vi "SA40144C.20201230 Data Analysis.vi"() -> ()   [LabVIEW 2020]
uses:
  <vilib>/Analysis/baseanly.llb/Mean (DBL).vi
  <userlib>/_OpenG.lib/file/file.llb/Build Path - Traditional__ogtk.vi
  <userlib>/LevyLab/LV to ITX/Data/Data.lvclass
  <vilib>/Analysis/NI_AALBase.lvlib
  <userlib>/LevyLab/XY Utilities/xy_utilities.lvlib
panel:
  out "Temp vs t":T1(graph)
  in  "Update":bool
  in  "Temps to keep (Lifespan)":i32=26
  in  "Temps to keep (Arrhenius fit)":i32=26
  out "E_a":dbl[](array[numeric])
  in  "Trimming":i32=400
  out "G4T vs t  2D":T1(graph)
  out "G2T vs t 2D":T1(graph)
  in  "Data File":path=path "G:/My Drive/ansom/Data/PPMS 2/SA40144C.20201230/01 - Temp Sweep 1 HR/SA40144C.20201230.275K.dat"
  in  "Final Temp":i32=400
  in  "Temp Step":i32=5
  in  "Init Temp":i32=275
  in  "Source Voltage":dbl=0.01
  in  "OK":bool
  out "error out":errorcluster
  in  "error in (no error)":errorcluster
  out "G4T vs t":T1(graph)
  out "Arrhenius":T1(graph)
  out "Lifespan vs Temp (hrs)":cluster{i32[], dbl[]}[](graph)
  out "G2T vs t":T1(graph)
  # "2T"
  # "4T"
  # "2T 2D"
  # "4T 2D"
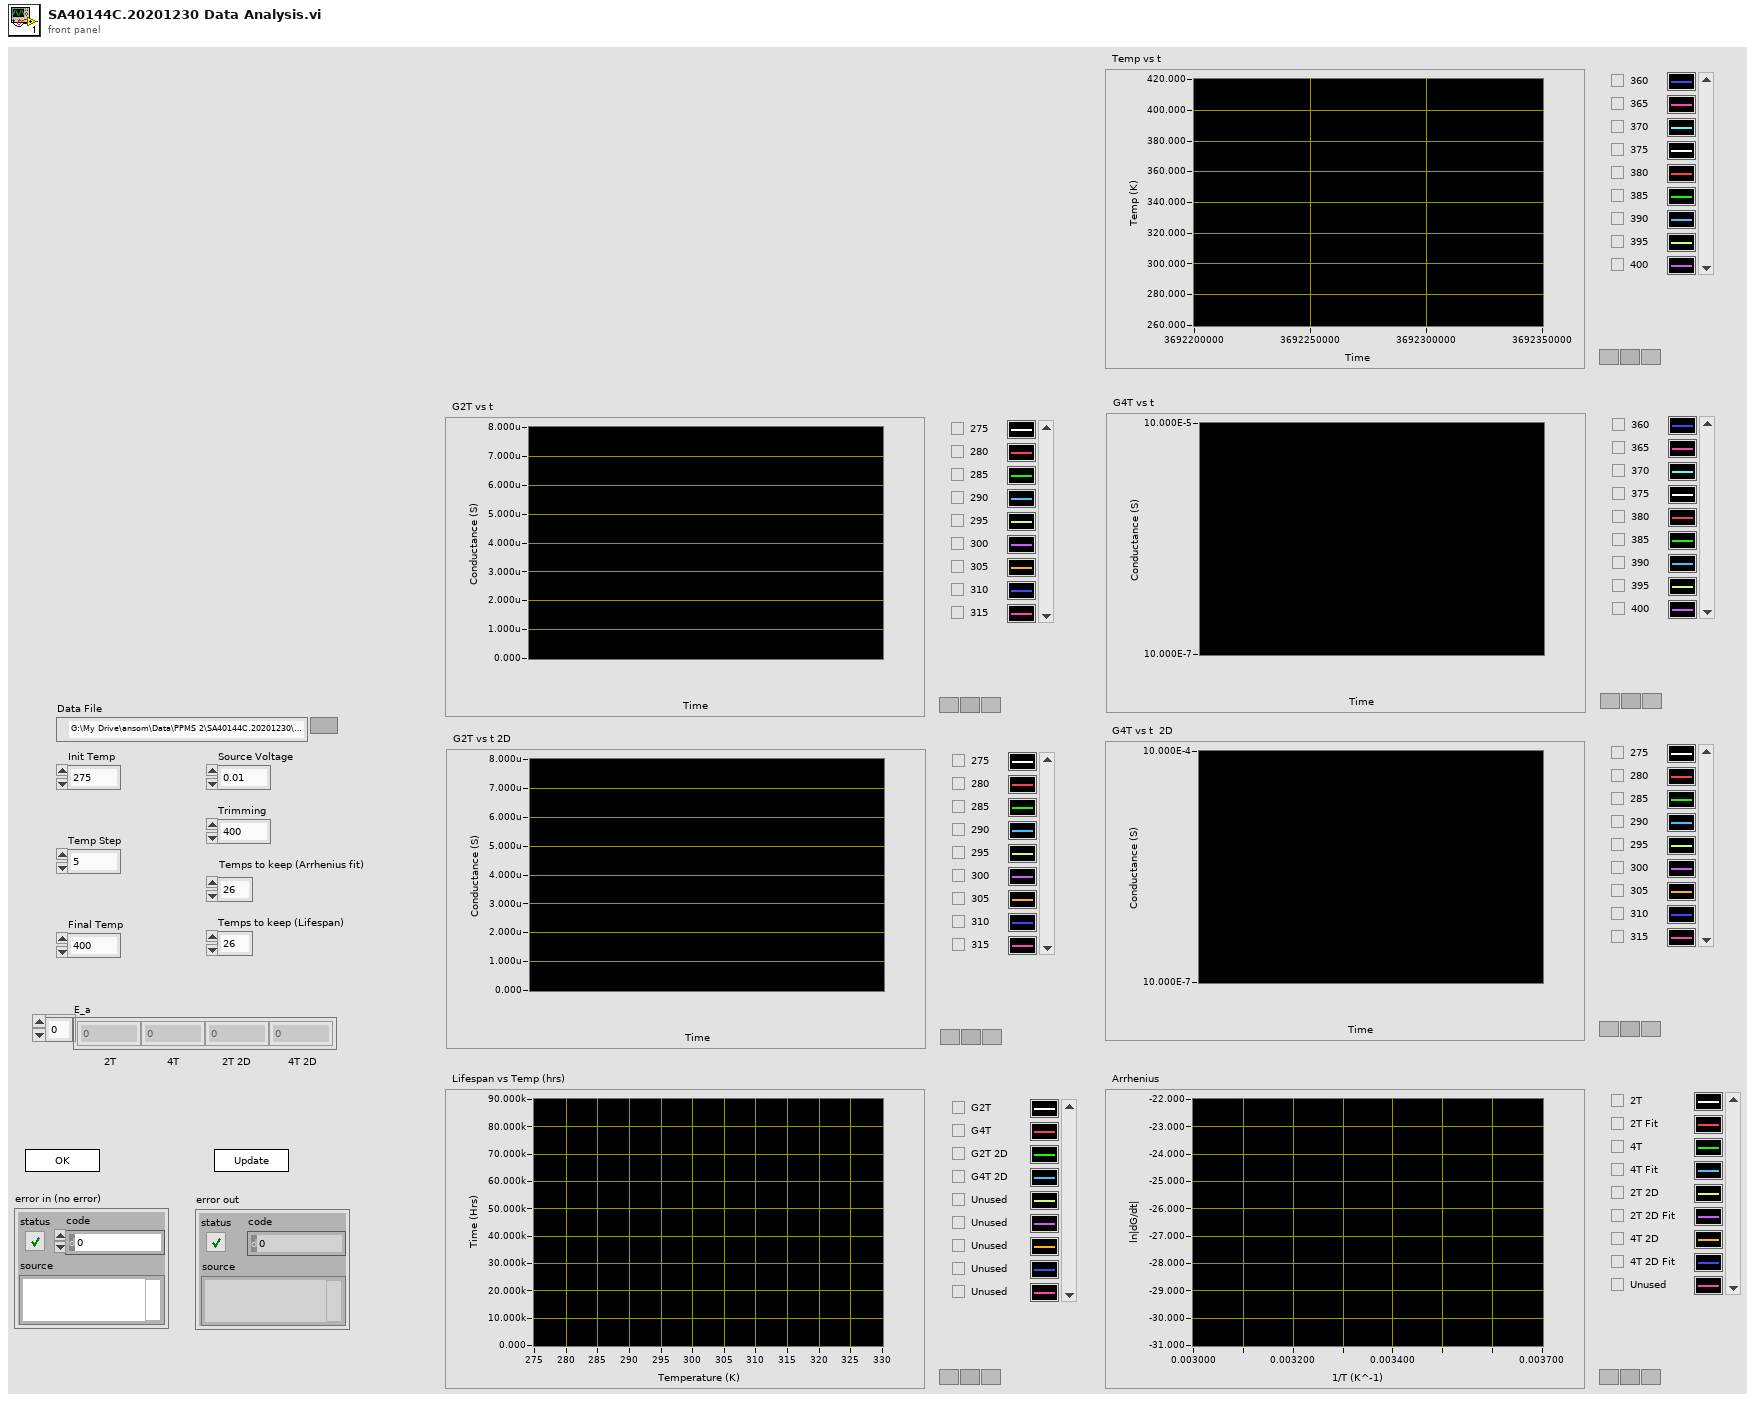
[diagram p1: front panel]
types:
  T1 = cluster{"Data":dbl[], "Best Exponential Fit":dbl[]}[]
  T2 = enum32{"Invalid", "Standard", "Closed", "Hidden", "Minimized", "Maximized"}
  T3 = enum32{"invalid app kind", "Development System", "Run Time System", "Student Edition", "Embedded LabVIEW", "Evaluation", "Custom"}
  T4 = cluster{"Core":cluster{"Current VI Reference":refnum<vi>, "Close Panel on Exit?":bool}, "G2T 1D":cluster{dbl[], dbl[]}[], "G4T 1D":cluster{dbl[], dbl[]}[], "G2T 2D":cluster{dbl[], dbl[]}[], "G4T 2D":cluster{dbl[], dbl[]}[], "Temp":cluster{dbl[], dbl[]}[], "Source Voltage":dbl, "Final Temp":i32, "Init Temp":i32, "Temp Step":i32, "Data File":path, "Trimming":i32}
  T5 = cluster{"Current VI Reference":refnum<vi>, "Close Panel on Exit?":bool}
  T6 = typedef "Data.lvclass/Dictionary--cluster.ctl" = cluster{"key":string, "value":variant}
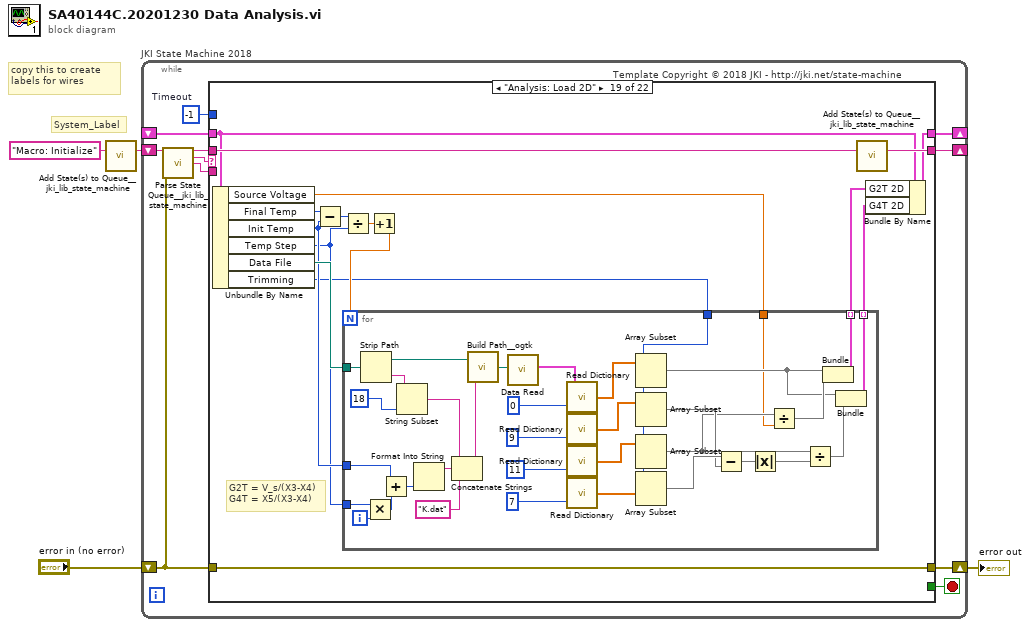
[diagram p0: block diagram]
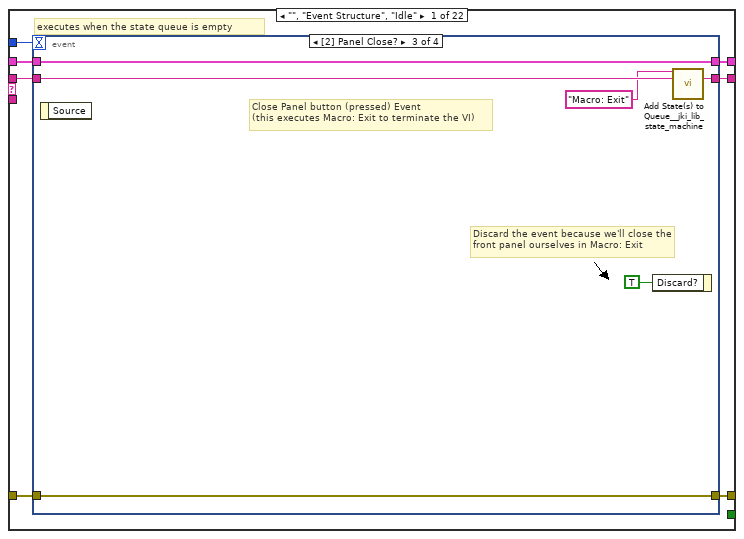
[diagram p2: hidden frame]
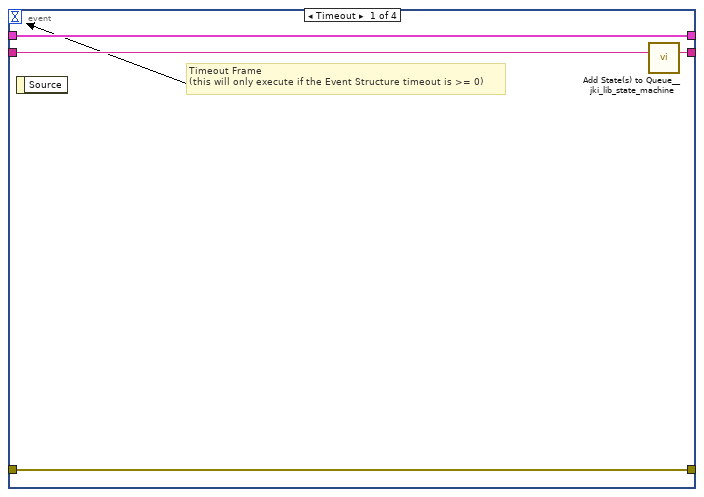
[diagram p3: hidden frame]
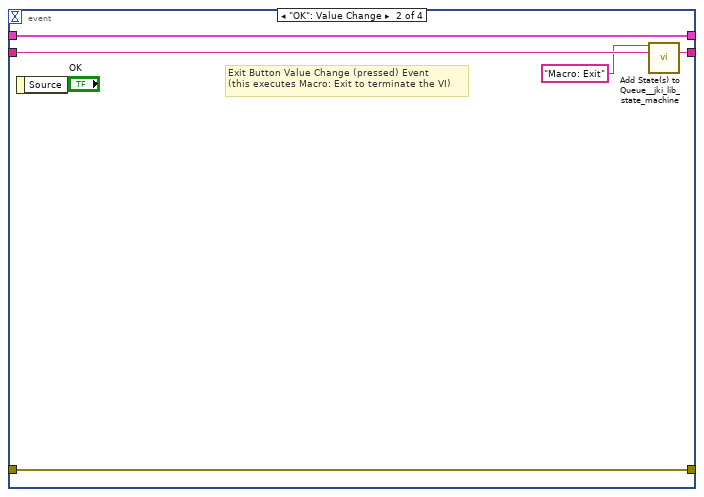
[diagram p4: hidden frame]
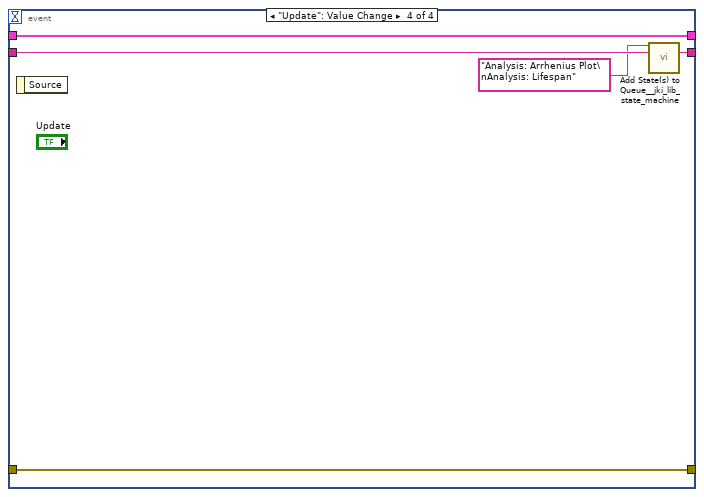
[diagram p5: hidden frame]
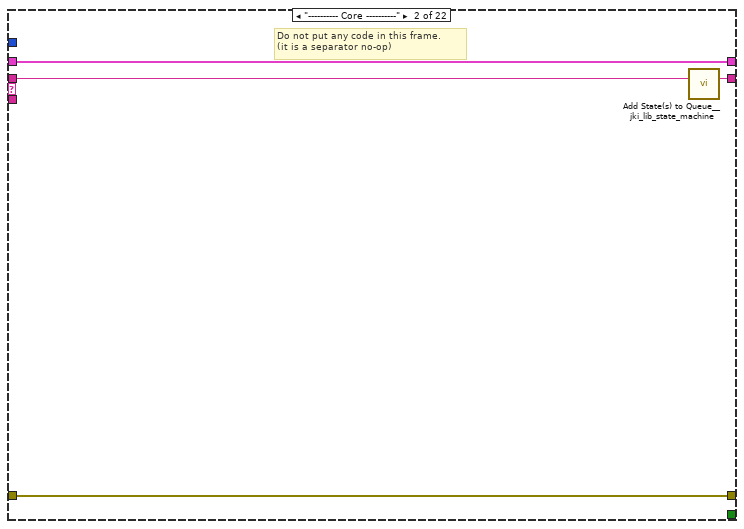
[diagram p6: hidden frame]
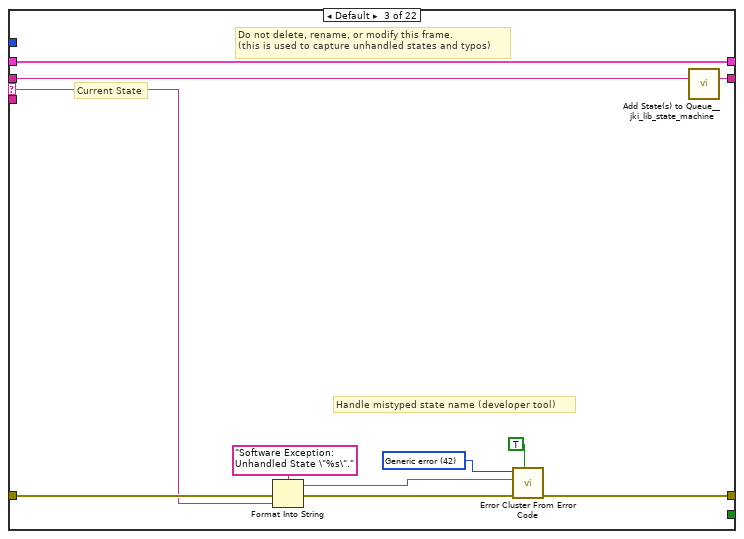
[diagram p7: hidden frame]
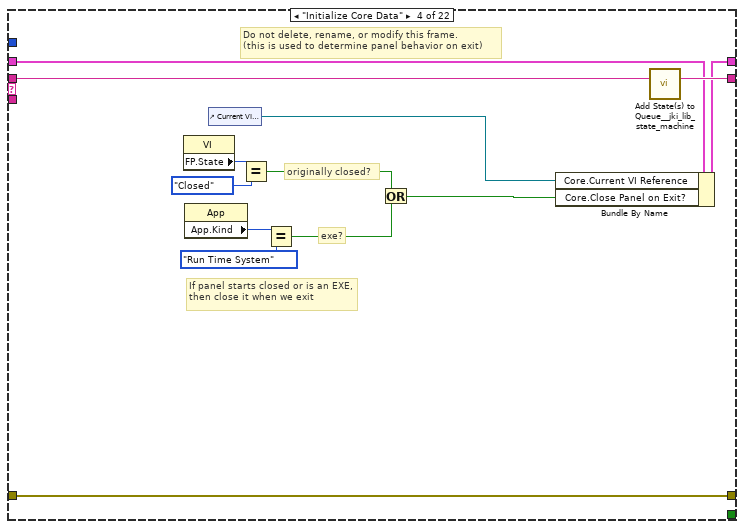
[diagram p8: hidden frame]
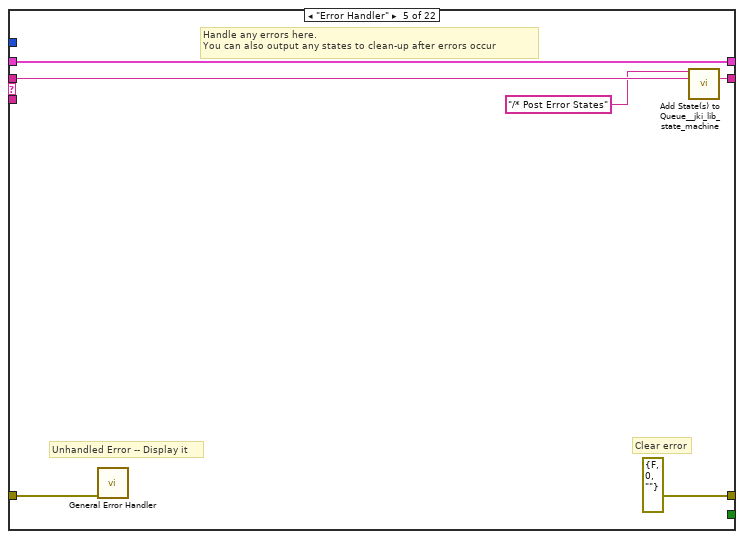
[diagram p9: hidden frame]
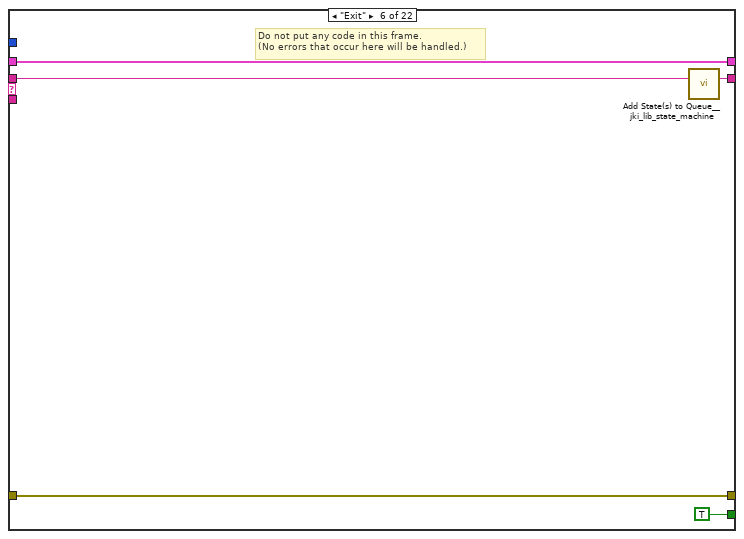
[diagram p10: hidden frame]
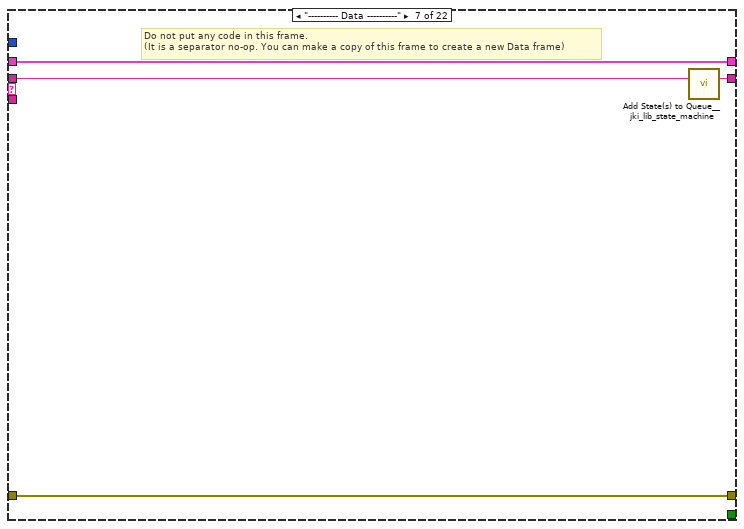
[diagram p11: hidden frame]
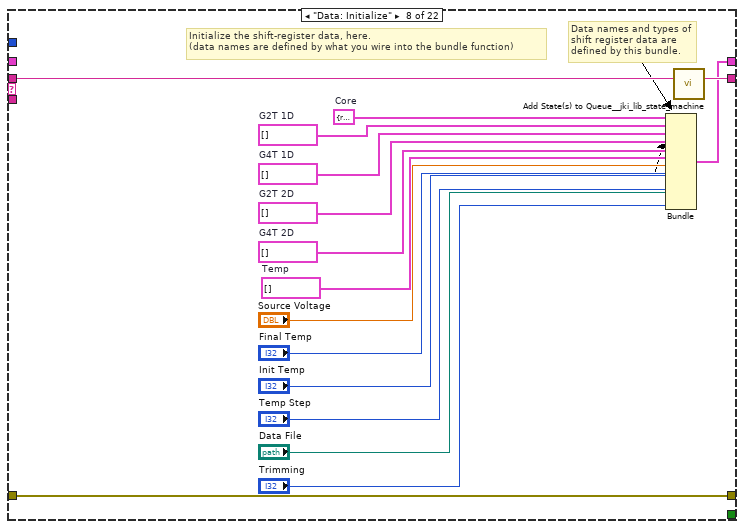
[diagram p12: hidden frame]
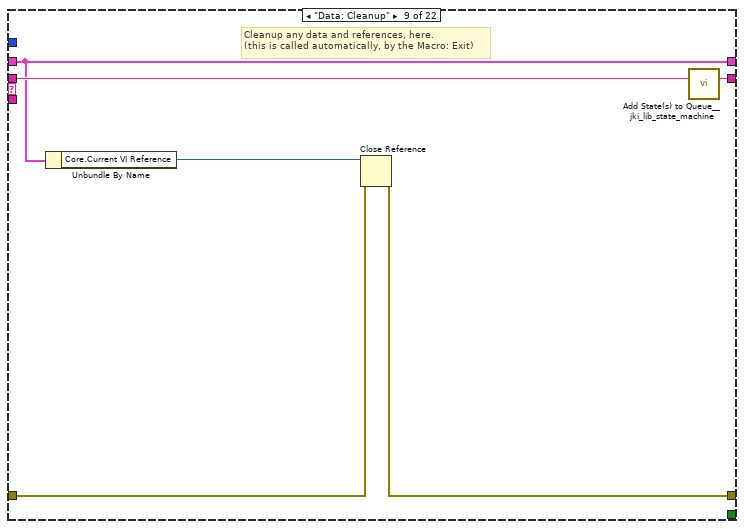
[diagram p13: hidden frame]
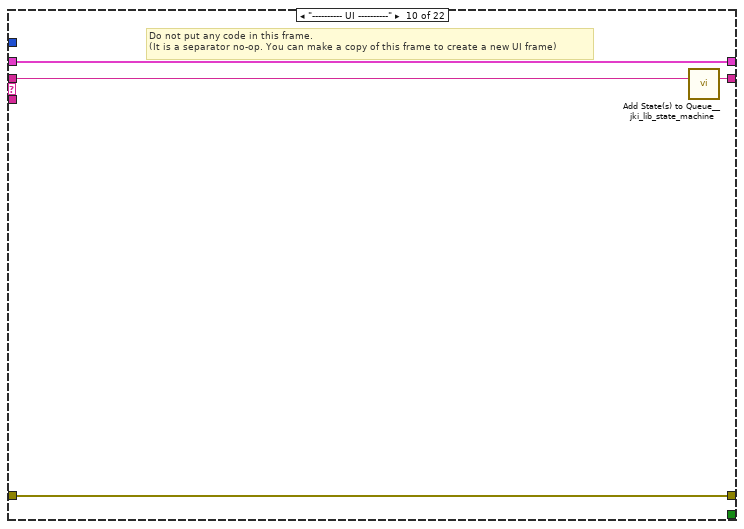
[diagram p14: hidden frame]
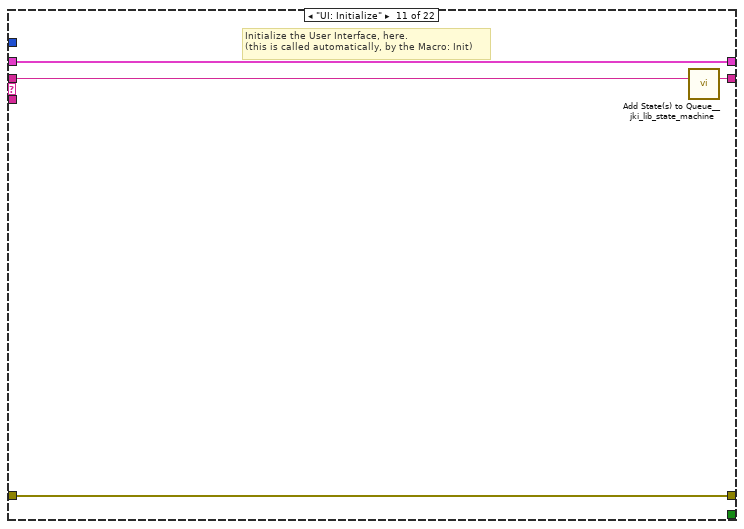
[diagram p15: hidden frame]
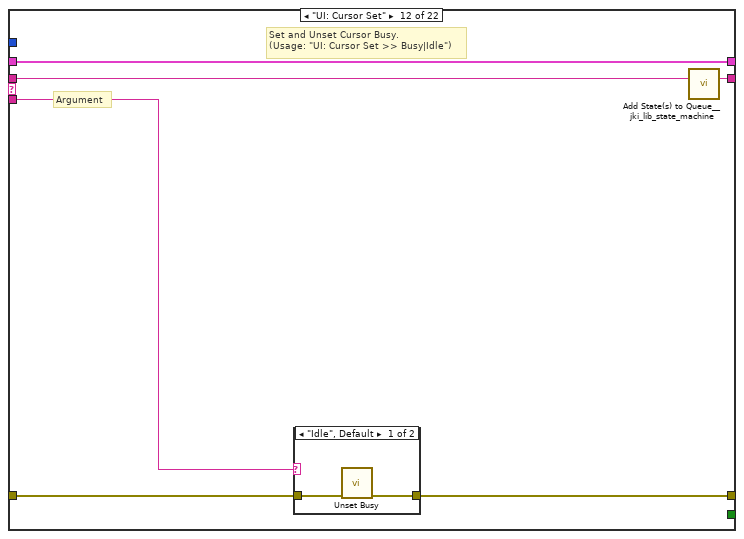
[diagram p16: hidden frame]
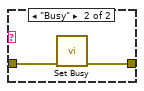
[diagram p17: hidden frame]
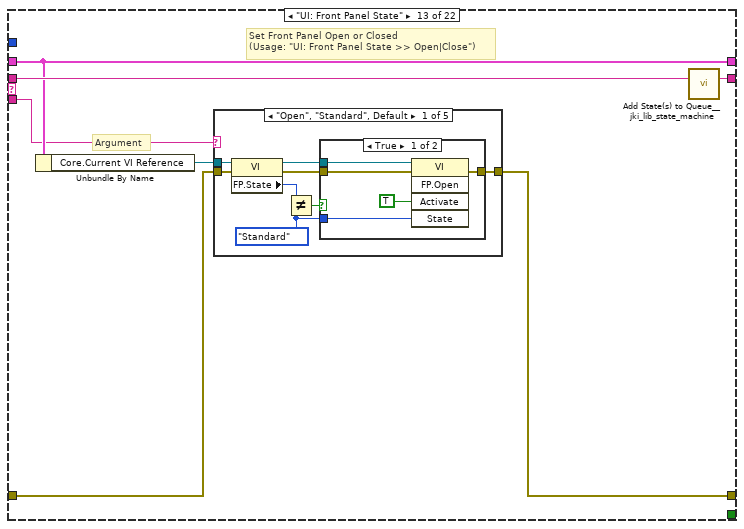
[diagram p18: hidden frame]
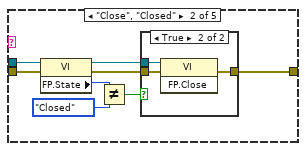
[diagram p20: hidden frame]
diagram:
  # "copy this to create labels for wires"
  # "System_Label"
  n1 = call <vilib>:"Add State(s) to Queue__jki_lib_state_machine.vi"("State(s) in (\"\")"="Macro: Initialize") -> ("States Out"=w4:string)  [unwired: 14 in]
  n2 = while "JKI State Machine 2018" {
    shift-right: [w8] -> _
    shift-left: _ -> [w7]
    shift-right: [w11] -> w1
    shift-left: "error in (no error)" -> [w5]
    shift-right: [w10] -> _
    shift-left: w4 -> [w12]
    stop <- w9 stop-if-true
    w6 = -1  # Timeout
    # "Template Copyright © 2018 JKI - http://jki.net/state-machine"
    n3 = call <vilib>:"Parse State Queue__jki_lib_state_machine.vi"("State Queue"=w12, "Error In (no error)"=w5) -> ("Remaining States"=w14:string, "Current State"=w15:string, "Arguments"=w13:string)  [unwired: 11 in]
    n4 = case shown="\"Analysis: Load 2D\"" w15 {
      selector: w15 -> [_ _ w47 _ _ _ _ _ _ _ _ _ _ _ _ _ _ _ _ _ _ _]
      tunnel: w14 -> [w22 w46 w51 w70 w76 w81 w85 w101 w107 w111 w115 w121 w132 w201 w206 w216 w220 w237 w292 w336 w380 w437]
      tunnel: w13 -> [_ _ _ _ _ _ _ _ _ _ _ w116 w126 _ _ _ _ _ _ _ _ _]
      tunnel: w7 -> [w20 w43 w49 w63 w73 w79 w82 _ w102 w108 w113 w119 w128 w198 w203 w213 w217 w231 w277 w333 w377 w417]
      tunnel: [w19 w44 w53 w67 errorcluster {"status"=FALSE, "code"=0, "source"=""} ("error out") w78 w83 w98 w103 w109 w112 w117 w129 w199 w204 w214 w218 w233 w290 w334 w378 w435] -> w11
      tunnel: w5 -> [w18 w44 w52 w67 w72 w78 w83 w98 w104 w109 w112 w118 w130 w199 w204 w214 w218 w233 w290 w334 w378 w435]
      tunnel: [w21 w45 w50 w69 w75 w80 w84 w100 w106 w110 w114 w120 w131 w200 w205 w215 w219 w236 w291 w335 w379 w436] -> w10
      tunnel: [_ _ _ _ _ TRUE _ _ _ _ _ _ _ _ _ _ _ _ _ _ _ _] -> w9
      tunnel: [w17 w43 w49 w68 w73 w79 w82 w99 w102 w108 w113 w119 w128 w198 w203 w213 w217 w232 w278 w333 w377 w417] -> w8
      tunnel: w6 -> [w16 _ _ _ _ _ _ _ _ _ _ _ _ _ _ _ _ _ _ _ _ _]
      frame "", "Event Structure", "Idle" {
        # "executes when the state queue is empty"
        n5 = event shown="[2] Panel Close?" {
          selector: _ -> [_ _ _ _]
          dyn-events: _ -> [_ _ _ _]
          timeout: w16 -> [_ _ _ _]
          tunnel: w22 -> [w26 w31 w37 w41]
          tunnel: [w25 w30 w36 w40] -> w21
          tunnel: w20 -> [w23 w28 w34 w42]
          tunnel: [w24 w29 w35 w38] -> w19
          tunnel: w18 -> [w24 w29 w35 w38]
          tunnel: [w23 w28 w34 w42] -> w17
          event Timeout {
            # "Timeout Frame\n(this will only execute if the Event Structure timeout is >= 0)"
            n6 = event-data() -> ()  [unwired: 1 in, 1 out]
            n7 = call <vilib>:"Add State(s) to Queue__jki_lib_state_machine.vi"("State(s) in (\"\")"=w26) -> ("States Out"=w25:string)  [unwired: 14 in]
          }
          event "OK": Value Change {
            # "Exit Button Value Change (pressed) Event\n(this executes Macro: Exit to terminate the VI)"
            n8 = event-data() -> ()  [unwired: 1 in, 1 out]
            n9 = call <vilib>:"Add State(s) to Queue__jki_lib_state_machine.vi"("State(s) in Front (\"\")"="Macro: Exit", "State(s) in (\"\")"=w31) -> ("States Out"=w30:string)  [unwired: 13 in]
          }
          event Panel Close? {
            # "Discard the event because we'll close the front panel ourselves in Macro: Exit"
            # "Close Panel button (pressed) Event\n(this executes Macro: Exit to terminate the VI)"
            n10 = event-data() -> ()  [unwired: 1 in, 1 out]
            n11 = event-data("Discard?"=TRUE) -> ()  [unwired: 1 in, 1 out]
            n12 = call <vilib>:"Add State(s) to Queue__jki_lib_state_machine.vi"("State(s) in Front (\"\")"="Macro: Exit", "State(s) in (\"\")"=w37) -> ("States Out"=w36:string)  [unwired: 13 in]
          }
          event "Update": Value Change {
            n13 = event-data() -> ()  [unwired: 1 in, 1 out]
            n14 = call <vilib>:"Add State(s) to Queue__jki_lib_state_machine.vi"("State(s) in Front (\"\")"="Analysis: Arrhenius Plot\nAnalysis: Lifespan" ("State(s) in Front (\"\")"), "State(s) in (\"\")"=w41) -> ("States Out"=w40:string)  [unwired: 13 in]
          }
        }
      }
      frame "---------- Core ----------" {
        # "Do not put any code in this frame.\n(it is a separator no-op)"
        n15 = call <vilib>:"Add State(s) to Queue__jki_lib_state_machine.vi"("State(s) in (\"\")"=w46) -> ("States Out"=w45:string)  [unwired: 14 in]
      }
      frame Default {
        w56 = 42 items=["No error", "Argument error", "Memory is full", "Out of zone", "End of file", "File already open", "Generic file I/O error", "File not found", "File permission error", "Disk is full", "Duplicate path", "Too many files open", "System feature not enabled", "Resource file not found", "Cannot add resource", "Resource not found", "Image not found", "Image memory error", "Pen does not exist", "Config type invalid", "Config token not found", "Config parse error", "Config memory error", "Bad external code format", "Bad external code offset", "External code not present", "Null window", "Destroy window error", "Null menu", "Print aborted", "Bad print record", "Print driver error", "Windows error during printing", "Memory error during printing", "Print dialog error", "Generic print error", "Invalid device refnum", "Device not found", "Device parameter error", "Device unit error", "Cannot open device", "Device call aborted", "Generic error", "Cancelled by user", "Object ID too low", "Object ID too high", "Object not in heap", "Unknown heap", "Unknown object (invalid DefProc)", "Unknown object (DefProc not in table)", "Message out of range", "Invalid (null) method", "Unknown message", "Manager call not supported", "Bad address", "Network operation in progress", "Network operation timed out", "Connection is busy", "Network attribute not supported", "Network error", "Address in use", "System out of memory", "Connection aborted", "Connection refused", "Not connected", "Already connected", "Connection closed", "Initialization error (interapplication manager)", "Bad occurrence", "Wait on unbound occurrence handler", "Occurrence queue overflow", "Datalog type conflict", "Unused", "Unrecognized type (interapplication manager)", "Memory corrupt", "Failed to make temporary DLL", "Old CIN version", "Drag socket not found", "Failed to load drop-object", "Failed to register OLE object", "Failed to release OLE object", "Format specifier type mismatch", "Unknown format specifier", "Too few format specifiers", "Too many format specifiers", "Scan failed", "Newer CIN version", "Error converting to variant", "Runtime menu error", "Password tampered", "Variant attribute not found", "Incompatible variant data type", "Event data is not available", "Event Store is not present", "Occurrence is not found", "Event Queue is not created", "Event info is not available", "Refnum passed is NULL", "Error retrieving Class GUID", "Error retrieving CoClass GUID", "Error retrieving TypeLib GUID.", "Bad built application magic bytes.", "Specific driver is different from the specific driver associated with the Logical Name.", "There is no session opened to the class driver.", "Max Error", "MAX - Error with config objects", "MAX - Error loading configuration", "MAX - Group not supported"]
        # "Current State"
        # "Do not delete, rename, or modify this frame.\n(this is used to capture unhandled states and typos)"
        # "Handle mistyped state name (developer tool)"
        n16 = Format Into String(format string="Software Exception: Unhandled State \"%s\"." ("message"), error in=w52, w47) -> (resulting string=w55:string, error out=w54:errorcluster)  [unwired: 1 in]
        n17 = call <vilib>:"Error Cluster From Error Code.vi"("show call chain? (False)"=TRUE, "error in (no error)"=w54, "error message (\"\")"=w55, "error code (0)"=w56) -> ("error out"=w53:errorcluster)  [unwired: 5 in]
        n18 = call <vilib>:"Add State(s) to Queue__jki_lib_state_machine.vi"("State(s) in (\"\")"=w51) -> ("States Out"=w50:string)  [unwired: 14 in]
      }
      frame "Initialize Core Data" {
        # "Do not delete, rename, or modify this frame.\n(this is used to determine panel behavior on exit)"
        # "originally closed?"
        # "exe?"
        # "If panel starts closed or is an EXE, then close it when we exit"
        n19 = property class="VI"() -> ("FP.State"=w60:T2)  [unwired: 2 in, 2 out]
        n20 = property class="App"() -> ("App.Kind"=w66:T3)  [unwired: 2 in, 2 out]
        n21 = control-ref of="Current VI Reference"() -> (w61:refnum<vi>)
        n22 = Equal?(x=w60, y=T2."Closed" ("Front Panel Window:State")) -> (x = y?=w58:bool)
        n23 = Equal?(x=w66, y=T3."Run Time System" ("Application:Kind")) -> (x = y?=w64:bool)
        n24 = Or(x=w58, y=w64) -> (x .or. y?=w62:bool)
        n25 = Bundle By Name(cluster=w63, "Core.Current VI Reference"=w61, "Core.Close Panel on Exit?"=w62) -> (w68:T4)
        n26 = call <vilib>:"Add State(s) to Queue__jki_lib_state_machine.vi"("State(s) in (\"\")"=w70) -> ("States Out"=w69:string)  [unwired: 14 in]
      }
      frame "Error Handler" {
        # "Unhandled Error -- Display it"
        # "Handle any errors here.\nYou can also output any states to clean-up after errors occur"
        # "Clear error"
        n27 = call <vilib>:"General Error Handler.vi"("error in (no error)"=w72) -> ()  [unwired: 10 in, 5 out]
        n28 = call <vilib>:"Add State(s) to Queue__jki_lib_state_machine.vi"("State(s) in Front (\"\")"="/* Post Error States", "State(s) in (\"\")"=w76) -> ("States Out"=w75:string)  [unwired: 13 in]
      }
      frame "Exit" {
        # "Do not put any code in this frame.\n(No errors that occur here will be handled.)"
        n29 = call <vilib>:"Add State(s) to Queue__jki_lib_state_machine.vi"("State(s) in (\"\")"=w81) -> ("States Out"=w80:string)  [unwired: 14 in]
      }
      frame "---------- Data ----------" {
        # "Do not put any code in this frame.\n(It is a separator no-op. You can make a copy of this frame to create a new Data frame)"
        n30 = call <vilib>:"Add State(s) to Queue__jki_lib_state_machine.vi"("State(s) in (\"\")"=w85) -> ("States Out"=w84:string)  [unwired: 14 in]
      }
      frame "Data: Initialize" {
        w86 = cluster{dbl[], dbl[]}[] []  # Temp
        w95 = cluster{dbl[], dbl[]}[] []  # G4T 2D
        w94 = cluster{dbl[], dbl[]}[] []  # G2T 2D
        w93 = cluster{dbl[], dbl[]}[] []  # G4T 1D
        w92 = cluster{dbl[], dbl[]}[] []  # G2T 1D
        w97 = T5 {"Current VI Reference"=refnum, "Close Panel on Exit?"=FALSE}  # Core
        # "Data names and types of shift register data are defined by this bundle."
        # "Initialize the shift-register data, here.\n(data names are defined by what you wire into the bundle function)"
        n31 = Bundle("Core"=w97, "G2T 1D"=w92, "G4T 1D"=w93, "G2T 2D"=w94, "G4T 2D"=w95, "Temp"=w86, "Source Voltage"="Source Voltage", "Final Temp"="Final Temp", "Init Temp"="Init Temp", "Temp Step"="Temp Step", "Data File"="Data File", "Trimming"="Trimming") -> (w99:T4)  [unwired: 1 in]
        n32 = call <vilib>:"Add State(s) to Queue__jki_lib_state_machine.vi"("State(s) in (\"\")"=w101) -> ("States Out"=w100:string)  [unwired: 14 in]
      }
      frame "Data: Cleanup" {
        # "Cleanup any data and references, here.\n(this is called automatically, by the Macro: Exit)"
        n33 = Unbundle By Name(w102) -> ("Core.Current VI Reference"=w105:refnum<vi>)
        n34 = Close Reference(reference=w105, error in (no error)=w104) -> (error out=w103:errorcluster)
        n35 = call <vilib>:"Add State(s) to Queue__jki_lib_state_machine.vi"("State(s) in (\"\")"=w107) -> ("States Out"=w106:string)  [unwired: 14 in]
      }
      frame "---------- UI ----------" {
        # "Do not put any code in this frame.\n(It is a separator no-op. You can make a copy of this frame to create a new UI frame)"
        n36 = call <vilib>:"Add State(s) to Queue__jki_lib_state_machine.vi"("State(s) in (\"\")"=w111) -> ("States Out"=w110:string)  [unwired: 14 in]
      }
      frame "UI: Initialize" {
        # "Initialize the User Interface, here.\n(this is called automatically, by the Macro: Init)"
        n37 = call <vilib>:"Add State(s) to Queue__jki_lib_state_machine.vi"("State(s) in (\"\")"=w115) -> ("States Out"=w114:string)  [unwired: 14 in]
      }
      frame "UI: Cursor Set" {
        # "Argument"
        # "Set and Unset Cursor Busy.\n(Usage: \"UI: Cursor Set >> Busy|Idle\")"
        n38 = case shown="\"Idle\", Default" w116 {
          tunnel: w118 -> [w123 w125]
          tunnel: [w122 w124] -> w117
          frame "Idle", Default {
            n39 = call <vilib>:"Unset Busy.vi"("error in (no error)"=w123) -> ("error out"=w122:errorcluster)  [unwired: 10 in]
          }
          frame "Busy" {
            n40 = call <vilib>:"Set Busy.vi"("error in (no error)"=w125) -> ("error out"=w124:errorcluster)  [unwired: 9 in, 1 out]
          }
        }
        n41 = call <vilib>:"Add State(s) to Queue__jki_lib_state_machine.vi"("State(s) in (\"\")"=w121) -> ("States Out"=w120:string)  [unwired: 14 in]
      }
      frame "UI: Front Panel State" {
        # "Argument"
        # "Set Front Panel Open or Closed\n(Usage: \"UI: Front Panel State >> Open|Close\")"
        n42 = Unbundle By Name(w128) -> ("Core.Current VI Reference"=w127:refnum<vi>)
        n43 = case shown="\"Open\", \"Standard\", Default" w126 {
          tunnel: w130 -> [w138 w153 w164 w177 w190]
          tunnel: [w140 w154 w166 w179 w192] -> w129
          tunnel: w127 -> [w139 w151 w165 w178 w191]
          frame "Open", "Standard", Default {
            w133 = T2."Standard" ("State")
            n44 = property class="VI"(reference=w139, error in=w138) -> (reference out=w136:refnum<vi>, error out=w137:errorcluster, "FP.State"=w135:T2)
            n45 = Not Equal?(x=w135, y=w133) -> (x != y?=w134:bool)
            n46 = case shown="True" w134 {
              tunnel: [w144 w146] -> w140
              tunnel: w137 -> [w143 w146]
              tunnel: w136 -> [w142 _]
              tunnel: w133 -> [w141 _]
              frame True {
                n47 = invoke class="VI" method="FP.Open"(reference=w142, error in=w143, "Activate"=TRUE, "State"=w141) -> (error out=w144:errorcluster)  [unwired: 1 in, 4 out]
              }
              frame False {
              }
            }
          }
          frame "Close", "Closed" {
            n48 = property class="VI"(reference=w151, error in=w153) -> (reference out=w150:refnum<vi>, error out=w152:errorcluster, "FP.State"=w148:T2)
            n49 = Not Equal?(x=w148, y=T2."Closed" ("Front Panel Window:State")) -> (x != y?=w147:bool)
            n50 = case shown="True" w147 {
              tunnel: [w155 w158] -> w154
              tunnel: w152 -> [w155 w157]
              tunnel: w150 -> [_ w156]
              frame False {
              }
              frame True {
                n51 = invoke class="VI" method="FP.Close"(reference=w156, error in=w157) -> (error out=w158:errorcluster)  [unwired: 1 in, 2 out]
              }
            }
          }
          frame "Hidden", "Hide" {
            w159 = T2."Hidden" ("State")
            n52 = property class="VI"(reference=w165, error in=w164) -> (reference out=w162:refnum<vi>, error out=w163:errorcluster, "FP.State"=w161:T2)
            n53 = Not Equal?(x=w161, y=w159) -> (x != y?=w160:bool)
            n54 = case shown="True" w160 {
              tunnel: [w170 w171] -> w166
              tunnel: w163 -> [w169 w171]
              tunnel: w162 -> [w168 _]
              tunnel: w159 -> [w167 _]
              frame True {
                n55 = invoke class="VI" method="FP.Open"(reference=w168, error in=w169, "State"=w167) -> (error out=w170:errorcluster)  [unwired: 2 in, 4 out]
              }
              frame False {
              }
            }
          }
          frame "Minimize", "Minimized" {
            w172 = T2."Minimized" ("State")
            n56 = property class="VI"(reference=w178, error in=w177) -> (reference out=w175:refnum<vi>, error out=w176:errorcluster, "FP.State"=w174:T2)
            n57 = Not Equal?(x=w174, y=w172) -> (x != y?=w173:bool)
            n58 = case shown="True" w173 {
              tunnel: [w183 w184] -> w179
              tunnel: w176 -> [w182 w184]
              tunnel: w175 -> [w181 _]
              tunnel: w172 -> [w180 _]
              frame True {
                n59 = invoke class="VI" method="FP.Open"(reference=w181, error in=w182, "State"=w180) -> (error out=w183:errorcluster)  [unwired: 2 in, 4 out]
              }
              frame False {
              }
            }
          }
          frame "Maximize", "Maximized" {
            w185 = T2."Maximized" ("State")
            n60 = property class="VI"(reference=w191, error in=w190) -> (reference out=w188:refnum<vi>, error out=w189:errorcluster, "FP.State"=w187:T2)
            n61 = Not Equal?(x=w187, y=w185) -> (x != y?=w186:bool)
            n62 = case shown="True" w186 {
              tunnel: [w196 w197] -> w192
              tunnel: w189 -> [w195 w197]
              tunnel: w188 -> [w194 _]
              tunnel: w185 -> [w193 _]
              frame True {
                n63 = invoke class="VI" method="FP.Open"(reference=w194, error in=w195, "State"=w193) -> (error out=w196:errorcluster)  [unwired: 2 in, 4 out]
              }
              frame False {
              }
            }
          }
        }
        n64 = call <vilib>:"Add State(s) to Queue__jki_lib_state_machine.vi"("State(s) in (\"\")"=w132) -> ("States Out"=w131:string)  [unwired: 14 in]
      }
      frame "---------- Macro ----------" {
        # "Do not put any code in this frame.\n(It is a separator no-op. You can make a copy of this frame to create a new Macro frame)"
        n65 = call <vilib>:"Add State(s) to Queue__jki_lib_state_machine.vi"("State(s) in (\"\")"=w201) -> ("States Out"=w200:string)  [unwired: 14 in]
      }
      frame "Macro: Initialize" {
        # "Initialization Macro\n(This is called once, when the VI starts)"
        n66 = call <vilib>:"Add State(s) to Queue__jki_lib_state_machine.vi"("State(s) in Front (\"\")"="Data: Initialize\nInitialize Core Data\nUI: Initialize\nUI: Front Panel State >> Open\nAnalysis: Load 1D\nAnalysis: Load 2D\nAnalysis: Plot G vs t\nAnalysis: Arrhenius Plot\nAnalysis: Lifespan", "State(s) in (\"\")"=w206) -> ("States Out"=w205:string)  [unwired: 13 in]
      }
      frame "Macro: Exit" {
        # "Exit Macro\n(This is called once, when the VI exits)"
        n67 = Unbundle By Name(w213) -> ("Core.Close Panel on Exit?"=w212:bool)
        n68 = Select(t="UI: Front Panel State >> Close", s=w212, f="") -> (s? t:f=w209:string)
        n69 = call <vilib>:"Add State(s) to Queue__jki_lib_state_machine.vi"("State(s) in (\"\")"=w209, "State(s) at Back (\"\")"="Data: Cleanup\nExit") -> ("States Out"=w207:string)  [unwired: 13 in]
        n70 = call <vilib>:"Add State(s) to Queue__jki_lib_state_machine.vi"("State(s) in Front (\"\")"=w207, "State(s) in (\"\")"=w216) -> ("States Out"=w215:string)  [unwired: 13 in]
      }
      frame "---------- Analysis ----------" {
        # "Template Separator\n(You can make a copy of, or modify, this frame)"
        n71 = call <vilib>:"Add State(s) to Queue__jki_lib_state_machine.vi"("State(s) in (\"\")"=w220) -> ("States Out"=w219:string)  [unwired: 14 in]
      }
      frame "Analysis: Load 1D" {
        # "G2T = V_s/(X1-X7)\nG4T = X5/(X1-X7)"
        n72 = Unbundle By Name(w231) -> ("Source Voltage"=w230:dbl, "Final Temp"=w227:i32, "Init Temp"=w224:i32, "Temp Step"=w223:i32, "Data File"=w225:path, "Trimming"=w222:i32)
        n73 = Subtract(x=w227, y=w224) -> (x-y=w234:i32)
        n74 = Divide(x=w234, y=w223) -> (x/y=w235:dbl)
        n75 = Increment(x=w235) -> (x+1=w226:dbl)
        n76 = for {
          N: w226 -> [_]
          tunnel: w230 -> [w240]
          tunnel: [w262] -> w229 mode=indexing
          tunnel: [w261] -> w228 mode=indexing
          tunnel: w225 -> [w260]
          tunnel: w224 -> [w259]
          tunnel: w223 -> [w258]
          tunnel: w222 -> [w257]
          tunnel: [w252] -> w221 mode=indexing
          i -> [w267]
          n77 = Strip Path(path=w260) -> (stripped path=w272:path, name=w271:string)
          n78 = Multiply(x=w258, y=w267) -> (x*y=w268:i32)
          n79 = Add(x=w259, y=w268) -> (x+y=w273:i32)
          n80 = String Subset(string=w271, length (rest)=18) -> (substring=w269:string)  [unwired: 1 in]
          n81 = Format Into String(w273) -> (resulting string=w275:string)  [unwired: 3 in, 1 out]
          n82 = Concatenate Strings(w269, w275, "K.dat" ("string")) -> (w274:string)
          n83 = call-poly <userlib>:"Build Path__ogtk.vi"("name or relative path"=w274, "base path"=w272) -> ("appended path"=w276:path)
          n84 = call <userlib>:"Data Read.vi"("path"=w276) -> ("Data (Dictionary)"=w251:T6[])  [unwired: 7 in, 3 out]
          n85 = call "Read Dictionary.vi"("Numeric"=0, "Dictionary In"=w251) -> ("data"=w247:dbl[])
          n86 = call "Read Dictionary.vi"("Numeric"=3, "Dictionary In"=w251) -> ("data"=w241:dbl[])
          n87 = call "Read Dictionary.vi"("Numeric"=11 ("index"), "Dictionary In"=w251) -> ("data"=w242:dbl[])
          n88 = call "Read Dictionary.vi"("Numeric"=13, "Dictionary In"=w251) -> ("data"=w246:dbl[])
          n89 = call "Read Dictionary.vi"("Numeric"=1, "Dictionary In"=w251) -> ("data"=w245:dbl[])
          n90 = Array Subset(array=w247, index=w257) -> (w254:dbl[])  [unwired: 1 in]
          n91 = Array Subset(array=w241, index=w257) -> (w255:dbl[])  [unwired: 1 in]
          n92 = Array Subset(array=w242, index=w257) -> (w239:dbl[])  [unwired: 1 in]
          n93 = Array Subset(array=w246, index=w257) -> (w256:dbl[])  [unwired: 1 in]
          n94 = Subtract(x=w256, y=w255) -> (x-y=w266:dbl[])
          n95 = Absolute Value(x=w266) -> (abs(x)=w238:dbl[])
          n96 = Array Subset(array=w245) -> (w253:dbl[])  [unwired: 2 in]
          n97 = Divide(x=w239, y=w240) -> (x/y=w264:dbl[])
          n98 = Divide(x=w239, y=w238) -> (x/y=w265:dbl[])
          n99 = Bundle(w254, w264) -> (w262:cluster{dbl[], dbl[]})  [unwired: 1 in]
          n100 = Bundle(w254, w253) -> (w252:cluster{dbl[], dbl[]})  [unwired: 1 in]
          n101 = Bundle(w254, w265) -> (w261:cluster{dbl[], dbl[]})  [unwired: 1 in]
        }
        n102 = call <vilib>:"Add State(s) to Queue__jki_lib_state_machine.vi"("State(s) in (\"\")"=w237) -> ("States Out"=w236:string)  [unwired: 14 in]
        n103 = Bundle By Name(cluster=w231, "G2T 1D"=w229, "G4T 1D"=w228, "Temp"=w221) -> (w232:T4)
      }
      frame "Analysis: Load 2D" {
        # "G2T = V_s/(X3-X4)\nG4T = X5/(X3-X4)"
        n104 = Unbundle By Name(w277) -> ("Source Voltage"=w287:dbl, "Final Temp"=w284:i32, "Init Temp"=w281:i32, "Temp Step"=w280:i32, "Data File"=w282:path, "Trimming"=w279:i32)
        n105 = Subtract(x=w284, y=w281) -> (x-y=w288:i32)
        n106 = Divide(x=w288, y=w280) -> (x/y=w289:dbl)
        n107 = Increment(x=w289) -> (x+1=w283:dbl)
        n108 = for {
          N: w283 -> [_]
          tunnel: w287 -> [w294]
          tunnel: [w313] -> w286 mode=indexing
          tunnel: [w312] -> w285 mode=indexing
          tunnel: w282 -> [w311]
          tunnel: w281 -> [w310]
          tunnel: w280 -> [w309]
          tunnel: w279 -> [w308]
          i -> [w318]
          n109 = Strip Path(path=w311) -> (stripped path=w323:path, name=w322:string)
          n110 = Multiply(x=w309, y=w318) -> (x*y=w319:i32)
          n111 = Add(x=w310, y=w319) -> (x+y=w324:i32)
          n112 = String Subset(string=w322, length (rest)=18) -> (substring=w320:string)  [unwired: 1 in]
          n113 = Format Into String(w324) -> (resulting string=w326:string)  [unwired: 3 in, 1 out]
          n114 = Concatenate Strings(w320, w326, "K.dat" ("string")) -> (w325:string)
          n115 = call-poly <userlib>:"Build Path__ogtk.vi"("name or relative path"=w325, "base path"=w323) -> ("appended path"=w327:path)
          n116 = call <userlib>:"Data Read.vi"("path"=w327) -> ("Data (Dictionary)"=w304:T6[])  [unwired: 7 in, 3 out]
          n117 = call "Read Dictionary.vi"("Numeric"=0, "Dictionary In"=w304) -> ("data"=w303:dbl[])
          n118 = call "Read Dictionary.vi"("Numeric"=9, "Dictionary In"=w304) -> ("data"=w300:dbl[])
          n119 = call "Read Dictionary.vi"("Numeric"=11 ("index"), "Dictionary In"=w304) -> ("data"=w301:dbl[])
          n120 = call "Read Dictionary.vi"("Numeric"=7, "Dictionary In"=w304) -> ("data"=w302:dbl[])
          n121 = Array Subset(array=w303, index=w308) -> (w306:dbl[])  [unwired: 1 in]
          n122 = Array Subset(array=w300, index=w308) -> (w305:dbl[])  [unwired: 1 in]
          n123 = Array Subset(array=w301, index=w308) -> (w295:dbl[])  [unwired: 1 in]
          n124 = Array Subset(array=w302, index=w308) -> (w307:dbl[])  [unwired: 1 in]
          n125 = Subtract(x=w307, y=w305) -> (x-y=w317:dbl[])
          n126 = Absolute Value(x=w317) -> (abs(x)=w293:dbl[])
          n127 = Divide(x=w295, y=w294) -> (x/y=w315:dbl[])
          n128 = Divide(x=w295, y=w293) -> (x/y=w316:dbl[])
          n129 = Bundle(w306, w315) -> (w313:cluster{dbl[], dbl[]})  [unwired: 1 in]
          n130 = Bundle(w306, w316) -> (w312:cluster{dbl[], dbl[]})  [unwired: 1 in]
        }
        n131 = call <vilib>:"Add State(s) to Queue__jki_lib_state_machine.vi"("State(s) in (\"\")"=w292) -> ("States Out"=w291:string)  [unwired: 14 in]
        n132 = Bundle By Name(cluster=w277, "G2T 2D"=w286, "G4T 2D"=w285) -> (w278:T4)
      }
      frame "Analysis: Plot G vs t" {
        n133 = Unbundle By Name(w333) -> ("G2T 1D"=→"G2T vs t":cluster{dbl[], dbl[]}[], "G4T 1D"=→"G4T vs t":cluster{dbl[], dbl[]}[], "G2T 2D"=→"G2T vs t 2D":cluster{dbl[], dbl[]}[], "G4T 2D"=→"G4T vs t  2D":cluster{dbl[], dbl[]}[], "Temp"=→"Temp vs t":cluster{dbl[], dbl[]}[])
        n134 = call <vilib>:"Add State(s) to Queue__jki_lib_state_machine.vi"("State(s) in (\"\")"=w336) -> ("States Out"=w335:string)  [unwired: 14 in]
      }
      frame "Analysis: Arrhenius Plot" {
        n135 = Unbundle By Name(w377) -> ("G2T 1D"=w340:cluster{dbl[], dbl[]}[], "G4T 1D"=w339:cluster{dbl[], dbl[]}[], "G2T 2D"=w346:cluster{dbl[], dbl[]}[], "G4T 2D"=w348:cluster{dbl[], dbl[]}[], "Final Temp"=w374:i32, "Init Temp"=w372:i32, "Temp Step"=w371:i32)  [unwired: 1 out]
        n136 = Subtract(x=w374, y=w372) -> (x-y=w375:i32)
        n137 = Divide(x=w375, y=w371) -> (x/y=w376:dbl)
        n138 = Increment(x=w376) -> (x+1=w373:dbl)
        n139 = for {
          N: w373 -> [_]
          tunnel: w372 -> [w383]
          tunnel: w371 -> [w384]
          tunnel: [w381] -> w357 mode=indexing
          i -> [w385]
          n140 = Multiply(x=w384, y=w385) -> (x*y=w386:i32)
          n141 = Add(x=w383, y=w386) -> (x+y=w382:i32)
          n142 = Reciprocal(x=w382) -> (1/x=w381:dbl)
        }
        n143 = call-poly <userlib>:"Linear Fit.vi"("XY-data"=w340) -> ("slopes"=w337:dbl[])  [unwired: 4 in, 6 out]
        n144 = call-poly <userlib>:"Linear Fit.vi"("XY-data"=w339) -> ("slopes"=w338:dbl[])  [unwired: 4 in, 6 out]
        n145 = call-poly <userlib>:"Linear Fit.vi"("XY-data"=w346) -> ("slopes"=w345:dbl[])  [unwired: 4 in, 6 out]
        n146 = call-poly <userlib>:"Linear Fit.vi"("XY-data"=w348) -> ("slopes"=w347:dbl[])  [unwired: 4 in, 6 out]
        n147 = Absolute Value(x=w337) -> (abs(x)=w367:dbl[])
        n148 = Absolute Value(x=w338) -> (abs(x)=w368:dbl[])
        n149 = Absolute Value(x=w345) -> (abs(x)=w369:dbl[])
        n150 = Absolute Value(x=w347) -> (abs(x)=w370:dbl[])
        n151 = Natural Logarithm(1:w367) -> (0:w361:dbl[])
        n152 = Natural Logarithm(1:w368) -> (0:w360:dbl[])
        n153 = Natural Logarithm(1:w369) -> (0:w359:dbl[])
        n154 = Natural Logarithm(1:w370) -> (0:w358:dbl[])
        n155 = Array Subset(array=w361, length="Temps to keep (Arrhenius fit)") -> (w355:dbl[])  [unwired: 1 in]
        n156 = Array Subset(array=w360, length="Temps to keep (Arrhenius fit)") -> (w354:dbl[])  [unwired: 1 in]
        n157 = Array Subset(array=w359, length="Temps to keep (Arrhenius fit)") -> (w353:dbl[])  [unwired: 1 in]
        n158 = Array Subset(array=w358, length="Temps to keep (Arrhenius fit)") -> (w352:dbl[])  [unwired: 1 in]
        n159 = Array Subset(array=w357, length="Temps to keep (Arrhenius fit)") -> (w351:dbl[])  [unwired: 1 in]
        n160 = Bundle(w351, w355) -> (w364:cluster{dbl[], dbl[]})  [unwired: 1 in]
        n161 = Bundle(w351, w354) -> (w366:cluster{dbl[], dbl[]})  [unwired: 1 in]
        n162 = Bundle(w351, w353) -> (w365:cluster{dbl[], dbl[]})  [unwired: 1 in]
        n163 = Bundle(w351, w352) -> (w363:cluster{dbl[], dbl[]})  [unwired: 1 in]
        n164 = Build Array(w364, w366, w365, w363) -> (w344:cluster{dbl[], dbl[]}[])
        n165 = call-poly <userlib>:"Linear Fit.vi"("XY-data"=w344) -> ("Best Fits"=w343:cluster{"X-array":dbl[], "Y-array":dbl[]}[], "XY-data out"=w342:cluster{"X-array":dbl[], "Y-array":dbl[]}[], "slopes"=w341:dbl[])  [unwired: 4 in, 4 out]
        n166 = Multiply(x=w341, y=8.617333e-05) -> (x*y=→"E_a":dbl[])
        n167 = Interleave 1D Arrays(w342, w343) -> (→"Arrhenius":cluster{"X-array":dbl[], "Y-array":dbl[]}[])
        n168 = call <vilib>:"Add State(s) to Queue__jki_lib_state_machine.vi"("State(s) in (\"\")"=w380) -> ("States Out"=w379:string)  [unwired: 14 in]
      }
      frame "Analysis: Lifespan" {
        w395 = 3600
        # "Template Separator\n(You can make a copy of, or modify, this frame)"
        n169 = Unbundle By Name(w417) -> ("G2T 1D"=w434:cluster{dbl[], dbl[]}[], "G4T 1D"=w433:cluster{dbl[], dbl[]}[], "G2T 2D"=w432:cluster{dbl[], dbl[]}[], "G4T 2D"=w431:cluster{dbl[], dbl[]}[], "Final Temp"=w428:i32, "Init Temp"=w416:i32, "Temp Step"=w415:i32)  [unwired: 1 out]
        n170 = Subtract(x=w428, y=w416) -> (x-y=w429:i32)
        n171 = Divide(x=w429, y=w415) -> (x/y=w430:dbl)
        n172 = Increment(x=w430) -> (x+1=w414:dbl)
        n173 = for {
          N: w414 -> [_]
          tunnel: w416 -> [w452]
          tunnel: w415 -> [w451]
          tunnel: [w450] -> w413 mode=indexing
          i -> [w453]
          n174 = Multiply(x=w451, y=w453) -> (x*y=w454:i32)
          n175 = Add(x=w452, y=w454) -> (x+y=w450:i32)
        }
        n176 = call <userlib>:"Linear Fit (multiple).vi"("XY-data"=w434) -> ("XY-data out"=w408:cluster{"X-array":dbl[], "Y-array":dbl[]}[], "slopes"=w411:dbl[])  [unwired: 4 in, 5 out]
        n177 = call <userlib>:"Linear Fit (multiple).vi"("XY-data"=w433) -> ("XY-data out"=w407:cluster{"X-array":dbl[], "Y-array":dbl[]}[], "slopes"=w410:dbl[])  [unwired: 4 in, 5 out]
        n178 = call <userlib>:"Linear Fit (multiple).vi"("XY-data"=w432) -> ("XY-data out"=w406:cluster{"X-array":dbl[], "Y-array":dbl[]}[], "slopes"=w409:dbl[])  [unwired: 4 in, 5 out]
        n179 = call <userlib>:"Linear Fit (multiple).vi"("XY-data"=w431) -> ("XY-data out"=w405:cluster{"X-array":dbl[], "Y-array":dbl[]}[], "slopes"=w412:dbl[])  [unwired: 4 in, 5 out]
        n180 = for {
          tunnel: w408 -> [w446] mode=indexing
          tunnel: w407 -> [w447] mode=indexing
          tunnel: w406 -> [w448] mode=indexing
          tunnel: w405 -> [w449] mode=indexing
          tunnel: [w441] -> w404 mode=indexing
          tunnel: [w440] -> w403 mode=indexing
          tunnel: [w439] -> w402 mode=indexing
          tunnel: [w438] -> w401 mode=indexing
          n181 = Unbundle(w446) -> ("Y-array"=w442:dbl[])  [unwired: 1 out]
          n182 = Unbundle(w447) -> ("Y-array"=w443:dbl[])  [unwired: 1 out]
          n183 = Unbundle(w448) -> ("Y-array"=w444:dbl[])  [unwired: 1 out]
          n184 = Unbundle(w449) -> ("Y-array"=w445:dbl[])  [unwired: 1 out]
          n185 = call-poly <vilib>:"Mean.vi"("X"=w445) -> ("mean"=w438:dbl)  [unwired: 1 out]
          n186 = call-poly <vilib>:"Mean.vi"("X"=w444) -> ("mean"=w439:dbl)  [unwired: 1 out]
          n187 = call-poly <vilib>:"Mean.vi"("X"=w443) -> ("mean"=w440:dbl)  [unwired: 1 out]
          n188 = call-poly <vilib>:"Mean.vi"("X"=w442) -> ("mean"=w441:dbl)  [unwired: 1 out]
        }
        n189 = Divide(x=w404, y=w411) -> (x/y=w399:dbl[])
        n190 = Divide(x=w403, y=w410) -> (x/y=w398:dbl[])
        n191 = Divide(x=w402, y=w409) -> (x/y=w397:dbl[])
        n192 = Divide(x=w401, y=w412) -> (x/y=w396:dbl[])
        n193 = Divide(x=w399, y=w395) -> (x/y=w391:dbl[])
        n194 = Divide(x=w398, y=w395) -> (x/y=w392:dbl[])
        n195 = Divide(x=w397, y=w395) -> (x/y=w393:dbl[])
        n196 = Divide(x=w396, y=w395) -> (x/y=w394:dbl[])
        n197 = Array Subset(array=w391, length="Temps to keep (Lifespan)") -> (w422:dbl[])  [unwired: 1 in]
        n198 = Array Subset(array=w392, length="Temps to keep (Lifespan)") -> (w421:dbl[])  [unwired: 1 in]
        n199 = Array Subset(array=w393, length="Temps to keep (Lifespan)") -> (w420:dbl[])  [unwired: 1 in]
        n200 = Array Subset(array=w394, length="Temps to keep (Lifespan)") -> (w419:dbl[])  [unwired: 1 in]
        n201 = Array Subset(array=w413, length="Temps to keep (Lifespan)") -> (w418:i32[])  [unwired: 1 in]
        n202 = Absolute Value(x=w422) -> (abs(x)=w387:dbl[])
        n203 = Absolute Value(x=w421) -> (abs(x)=w388:dbl[])
        n204 = Absolute Value(x=w420) -> (abs(x)=w389:dbl[])
        n205 = Absolute Value(x=w419) -> (abs(x)=w390:dbl[])
        n206 = Bundle(w418, w387) -> (w425:cluster{i32[], dbl[]})  [unwired: 1 in]
        n207 = Bundle(w418, w388) -> (w427:cluster{i32[], dbl[]})  [unwired: 1 in]
        n208 = Bundle(w418, w389) -> (w426:cluster{i32[], dbl[]})  [unwired: 1 in]
        n209 = Bundle(w418, w390) -> (w424:cluster{i32[], dbl[]})  [unwired: 1 in]
        n210 = Build Array(w425, w427, w426, w424) -> (→"Lifespan vs Temp (hrs)":cluster{i32[], dbl[]}[])
        n211 = call <vilib>:"Add State(s) to Queue__jki_lib_state_machine.vi"("State(s) in (\"\")"=w437) -> ("States Out"=w436:string)  [unwired: 14 in]
      }
    }
  }
  "error out" <- w1
